vi "ControlMotorAbsMove.vi"(3 "是否需要进度":bool, 4 "运动模式":enum16{"轴向运动", "横向运动"}(ring), 5 "扫描坐标队列":refnum<queue>, 6 "轴向运动队列":refnum<queue>) -> (1 "是否到末位置":bool)   [LabVIEW 2018]
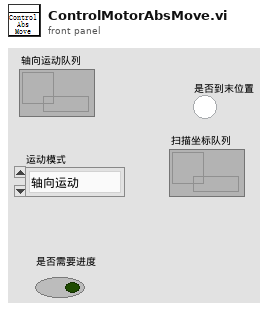
[diagram p1: front panel]
types:
  T1 = cluster{"电机":enum16{"Z", "Y", "X", "发散角", "俯仰", "旋转"}, "位置":dbl}
  T2 = cluster{"是否停止":enum16{"解除停止", "停止"}, "发生错误停止运行":enum16{"不停止", "停止"}, "发生错误退出运行":enum16{"不退出", "退出"}, "有效电平":cluster{"脉冲信号有效电平":enum16{"低电平有效", "高电平有效"}, "方向信号有效电平 ":enum16{"低电平有效", "高电平有效"}}, "运行脉宽":i32, "编码器使能":enum16{"不使能", "使能"}, "加速度和速度边界":cluster{"加速度最大":i32, "速度最大":i32}, "硬件限位设置":cluster{"正限位使能":enum16{"不使能", "使能"}, "正限位极性":enum16{"低电平有效", "高电平有效"}, "负限位使能 ":enum16{"不使能", "使能"}, "负限位极性 ":enum16{"低电平有效", "高电平有效"}}, "伺服报警":cluster{"伺服报警使能":enum16{"不使能", "使能"}, "伺服报警极性":enum16{"低电平有效", "高电平有效"}}, "电机使能":enum16{"不使能", "使能"}, "输出极性":cluster{"寄存器":u32, " fifo":u32, "Bit":u32, "输出极性控制":enum16{"脉冲+方向", "正负脉冲"}}, "运动模式":enum16{"普通模式", "跟踪模式"}, "加速度 puls/s2":i32, "运动速度":cluster{"峰值速度 puls/s":i32, "起始速度puls/s":i32}, "电机速度归一化常量":dbl}
  T3 = typedef "控制电机枚举器.ctl" = enum16{"Z", "Y", "X", "发散角", "俯仰", "旋转"}
  T4 = cluster{"控制电机":T3, "控制电机":T3, "单位mm":dbl, "单位mm":dbl}
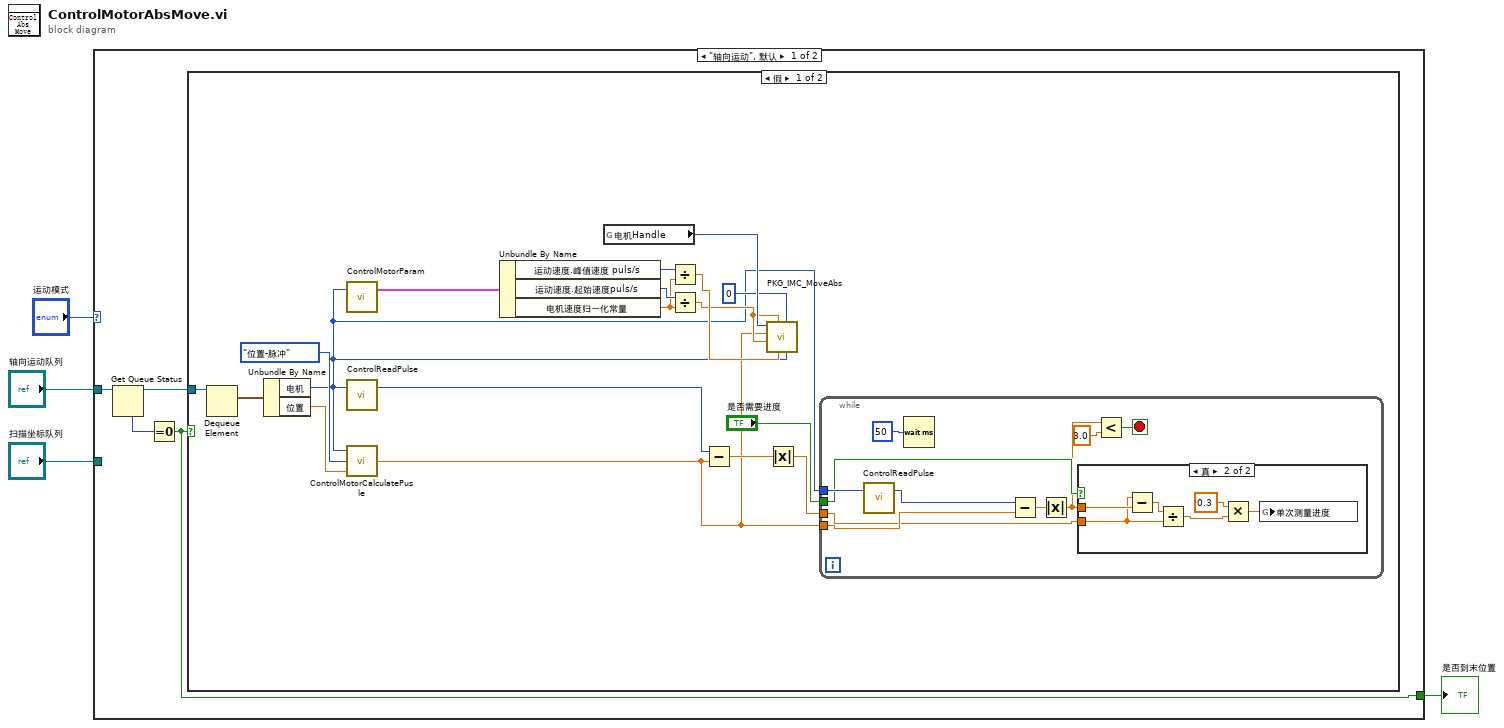
[diagram p0: block diagram]
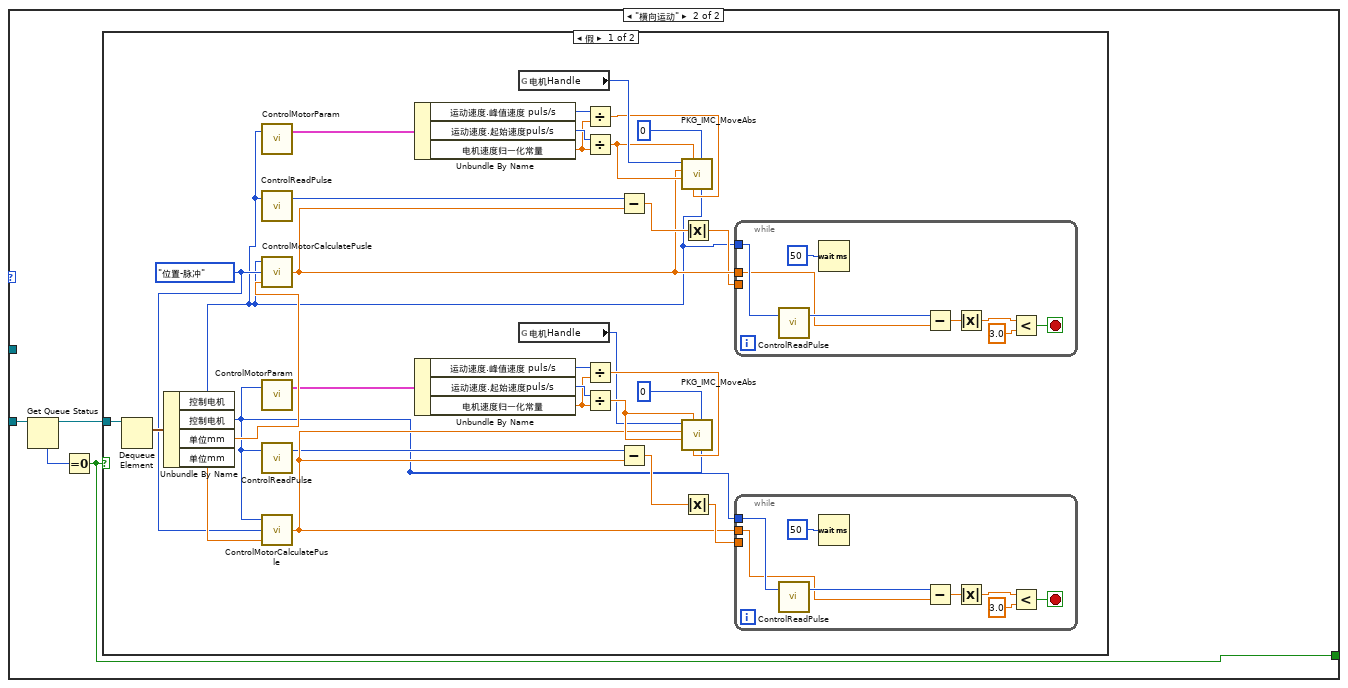
[diagram p4: hidden frame]
diagram:
  n1 = case shown="\"轴向运动\", 默认" "运动模式" {
    tunnel: [w7 w43] -> w4
    tunnel: "轴向运动队列" -> [w6 _]
    tunnel: "扫描坐标队列" -> [_ w44]
    frame "轴向运动", Default {
      n2 = Get Queue Status(queue=w6) -> (queue out=w5:refnum<queue>, # elements in queue=w8:i32)  [unwired: 2 in, 6 out]
      n3 = Equal To 0?(x=w8) -> (x = 0?=w7:bool)
      n4 = case shown="假" w7 {
        tunnel: w5 -> [w25 _]
        frame False {
          n5 = Dequeue Element(queue=w25) -> (element=w26:T1)  [unwired: 2 in, 3 out]
          n6 = Unbundle By Name(w26) -> ("电机"=w10:enum16{"Z", "Y", "X", "发散角", "俯仰", "旋转"}, "位置"=w24:dbl)
          n7 = call "ControlMotorParam.vi"("控制电机"=w10) -> ("轴电机参数输出"=w23:T2)  [unwired: 2 in]
          n8 = call "ControlReadPulse.vi"("控制电机"=w10) -> ("PulsOut"=w14:i32)  [unwired: 2 in]
          n9 = call "ControlMotorCalculatePusle.vi"("数据"=w24, "计算状态"=enum32{"位置-脉冲", "脉冲-位置"}."位置-脉冲", "控制电机"=w10) -> ("dataout"=w12:dbl)  [unwired: 2 in]
          n10 = Unbundle By Name(w23) -> ("运动速度.峰值速度 puls/s"=w21:i32, "运动速度.起始速度puls/s"=w19:i32, "电机速度归一化常量"=w18:dbl)
          n11 = global read "参数.vi" "电机Handle"() -> (w22:u32)
          n12 = Divide(x=w21, y=w18) -> (x/y=w20:dbl)
          n13 = Divide(x=w19, y=w18) -> (x/y=w17:dbl)
          n14 = Subtract(x=w14, y=w12) -> (x-y=w13:dbl)
          n15 = call "PKG_IMC_MoveAbs.vi"("axis"=w10, "wait"=0, "tgvel"=w20, "endvel"=w17, "startvel"=w17, "pos"=w12, "handle"=w22) -> ()  [unwired: 3 in, 2 out]
          n16 = Absolute Value(x=w13) -> (abs(x)=w11:dbl)
          n17 = while {
            tunnel: w10 -> [w35]
            tunnel: w12 -> [w33]
            tunnel: w11 -> [w28]
            tunnel: "是否需要进度" -> [w29]
            stop <- w30 stop-if-true
            n18 = call "ControlReadPulse.vi"("控制电机"=w35) -> ("PulsOut"=w34:i32)  [unwired: 2 in]
            n19 = Wait (ms)(milliseconds to wait=u32 50 ("等待时间（毫秒）")) -> ()  [unwired: 1 out]
            n20 = Subtract(x=w34, y=w33) -> (x-y=w32:dbl)
            n21 = Absolute Value(x=w32) -> (abs(x)=w27:dbl)
            n22 = case shown="真" w29 {
              tunnel: w28 -> [_ w40]
              tunnel: w27 -> [_ w42]
              frame False {
              }
              frame True {
                n23 = Subtract(x=w40, y=w42) -> (x-y=w41:dbl)
                n24 = Divide(x=w41, y=w40) -> (x/y=w39:dbl)
                n25 = Multiply(x=0.3, y=w39) -> (x*y=w37:dbl)
                n26 = global write "globalMessage.vi" "单次测量进度"(w37) -> ()
              }
            }
            n27 = Less?(x=w27, y=3.0) -> (x < y?=w30:bool)
          }
        }
        frame True {
        }
      }
    }
    frame "横向运动" {
      n28 = Get Queue Status(queue=w44) -> (queue out=w45:refnum<queue>, # elements in queue=w46:i32)  [unwired: 2 in, 6 out]
      n29 = Equal To 0?(x=w46) -> (x = 0?=w43:bool)
      n30 = case shown="假" w43 {
        tunnel: w45 -> [w76 _]
        frame False {
          w62 = enum32{"位置-脉冲", "脉冲-位置"}."位置-脉冲" ("计算状态")
          n31 = Dequeue Element(queue=w76) -> (element=w77:T4)  [unwired: 2 in, 3 out]
          n32 = Unbundle By Name(w77) -> ("控制电机"=w48:T3, "控制电机"=w47:T3, "单位mm"=w75:dbl, "单位mm"=w63:dbl)
          n33 = call "ControlMotorParam.vi"("控制电机"=w48) -> ("轴电机参数输出"=w74:T2)  [unwired: 2 in]
          n34 = call "ControlReadPulse.vi"("控制电机"=w48) -> ("PulsOut"=w51:i32)  [unwired: 2 in]
          n35 = call "ControlMotorCalculatePusle.vi"("数据"=w75, "计算状态"=w62, "控制电机"=w48) -> ("dataout"=w65:dbl)  [unwired: 2 in]
          n36 = call "ControlMotorParam.vi"("控制电机"=w47) -> ("轴电机参数输出"=w55:T2)  [unwired: 2 in]
          n37 = call "ControlReadPulse.vi"("控制电机"=w47) -> ("PulsOut"=w49:i32)  [unwired: 2 in]
          n38 = call "ControlMotorCalculatePusle.vi"("数据"=w63, "计算状态"=w62, "控制电机"=w47) -> ("dataout"=w50:dbl)  [unwired: 2 in]
          n39 = Unbundle By Name(w74) -> ("运动速度.峰值速度 puls/s"=w72:i32, "运动速度.起始速度puls/s"=w70:i32, "电机速度归一化常量"=w69:dbl)
          n40 = Unbundle By Name(w55) -> ("运动速度.峰值速度 puls/s"=w61:i32, "运动速度.起始速度puls/s"=w59:i32, "电机速度归一化常量"=w58:dbl)
          n41 = global read "参数.vi" "电机Handle"() -> (w73:u32)
          n42 = global read "参数.vi" "电机Handle"() -> (w54:u32)
          n43 = Divide(x=w72, y=w69) -> (x/y=w71:dbl)
          n44 = Divide(x=w70, y=w69) -> (x/y=w68:dbl)
          n45 = Divide(x=w61, y=w58) -> (x/y=w60:dbl)
          n46 = Divide(x=w59, y=w58) -> (x/y=w57:dbl)
          n47 = Subtract(x=w51, y=w65) -> (x-y=w66:dbl)
          n48 = Subtract(x=w49, y=w50) -> (x-y=w53:dbl)
          n49 = call "PKG_IMC_MoveAbs.vi"("axis"=w48, "wait"=0, "tgvel"=w71, "endvel"=w68, "startvel"=w68, "pos"=w65, "handle"=w73) -> ()  [unwired: 3 in, 2 out]
          n50 = call "PKG_IMC_MoveAbs.vi"("axis"=w47, "wait"=0, "tgvel"=w60, "endvel"=w57, "startvel"=w57, "pos"=w50, "handle"=w54) -> ()  [unwired: 3 in, 2 out]
          n51 = Absolute Value(x=w66) -> (abs(x)=w64:dbl)
          n52 = Absolute Value(x=w53) -> (abs(x)=w52:dbl)
          n53 = while {
            tunnel: w48 -> [w92]
            tunnel: w65 -> [w90]
            tunnel: w64 -> [_]
            stop <- w86 stop-if-true
            n54 = call "ControlReadPulse.vi"("控制电机"=w92) -> ("PulsOut"=w91:i32)  [unwired: 2 in]
            n55 = Wait (ms)(milliseconds to wait=u32 50 ("等待时间（毫秒）")) -> ()  [unwired: 1 out]
            n56 = Subtract(x=w91, y=w90) -> (x-y=w89:dbl)
            n57 = Absolute Value(x=w89) -> (abs(x)=w88:dbl)
            n58 = Less?(x=w88, y=3.0) -> (x < y?=w86:bool)
          }
          n59 = while {
            tunnel: w47 -> [w84]
            tunnel: w50 -> [w82]
            tunnel: w52 -> [_]
            stop <- w78 stop-if-true
            n60 = call "ControlReadPulse.vi"("控制电机"=w84) -> ("PulsOut"=w83:i32)  [unwired: 2 in]
            n61 = Wait (ms)(milliseconds to wait=u32 50 ("等待时间（毫秒）")) -> ()  [unwired: 1 out]
            n62 = Subtract(x=w83, y=w82) -> (x-y=w81:dbl)
            n63 = Absolute Value(x=w81) -> (abs(x)=w80:dbl)
            n64 = Less?(x=w80, y=3.0) -> (x < y?=w78:bool)
          }
        }
        frame True {
        }
      }
    }
  }
  "是否到末位置" <- w4
